vi "ToGraphML.vi"(8 "error in (no error)":errorcluster, 11 "SudokuState in":refnum<class "SudokuState.lvclass">) -> (0 "error out":errorcluster, 3 "SudokuState out":refnum<class "SudokuState.lvclass">)   [LabVIEW 2010, in "SudokuState.lvclass"]
uses:
  SudokuState.lvclass
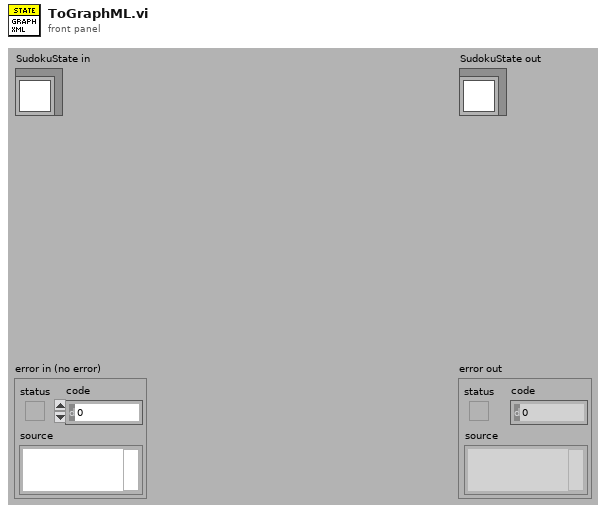
[diagram p1: front panel]
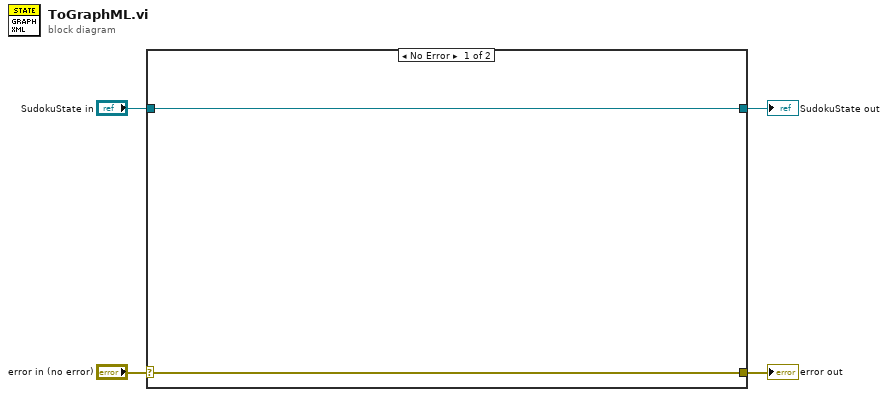
[diagram p0: block diagram]
diagram:
  n1 = case shown="No Error" "error in (no error)" {
    selector: "error in (no error)" -> [w6 w8]
    tunnel: [w6 w8] -> w3
    tunnel: [w5 w7] -> w1
    tunnel: "SudokuState in" -> [w5 w7]
    frame No Error {
    }
    frame Error {
    }
  }
  "error out" <- w3
  "SudokuState out" <- w1
